vi "TangensFilter3.vi"(4 "error IN":errorcluster, 5 "Max Angle REVERSE Disp":dbl, 6 "Max Angle FORWARD Displ":dbl, 7 "Finded Chains (X,Y,dX,dY)":dbl[][](array[numeric])) -> (0 "error out":errorcluster, 1 "Filtered Chains (X,Y,dX,dY)":dbl[][](array[numeric]), 2 "Saved Chains":i32, 3 "Angles OUT":dbl[][](array[numeric]))   [LabVIEW 2013]
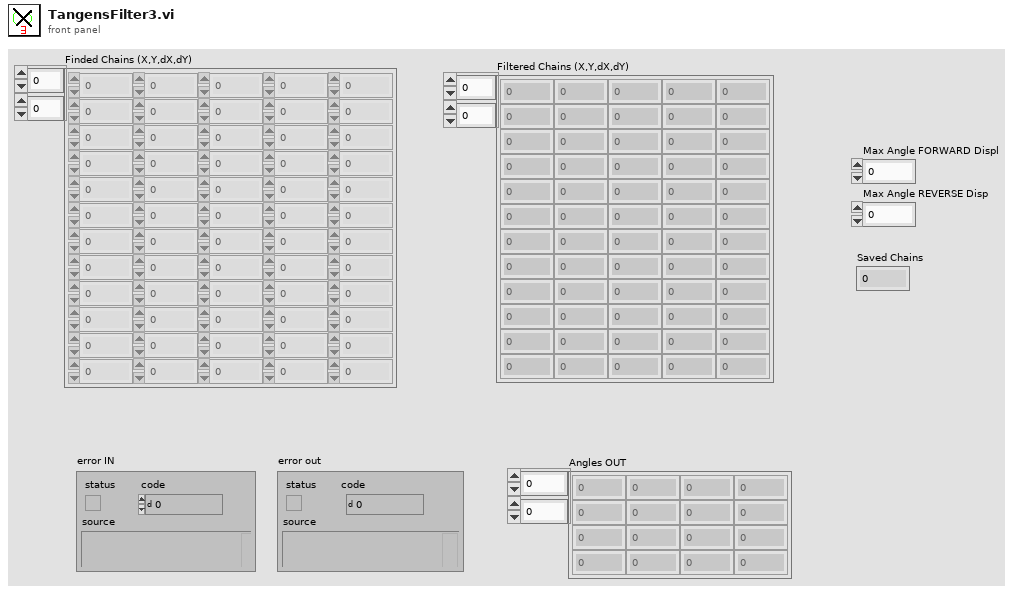
[diagram p1: front panel]
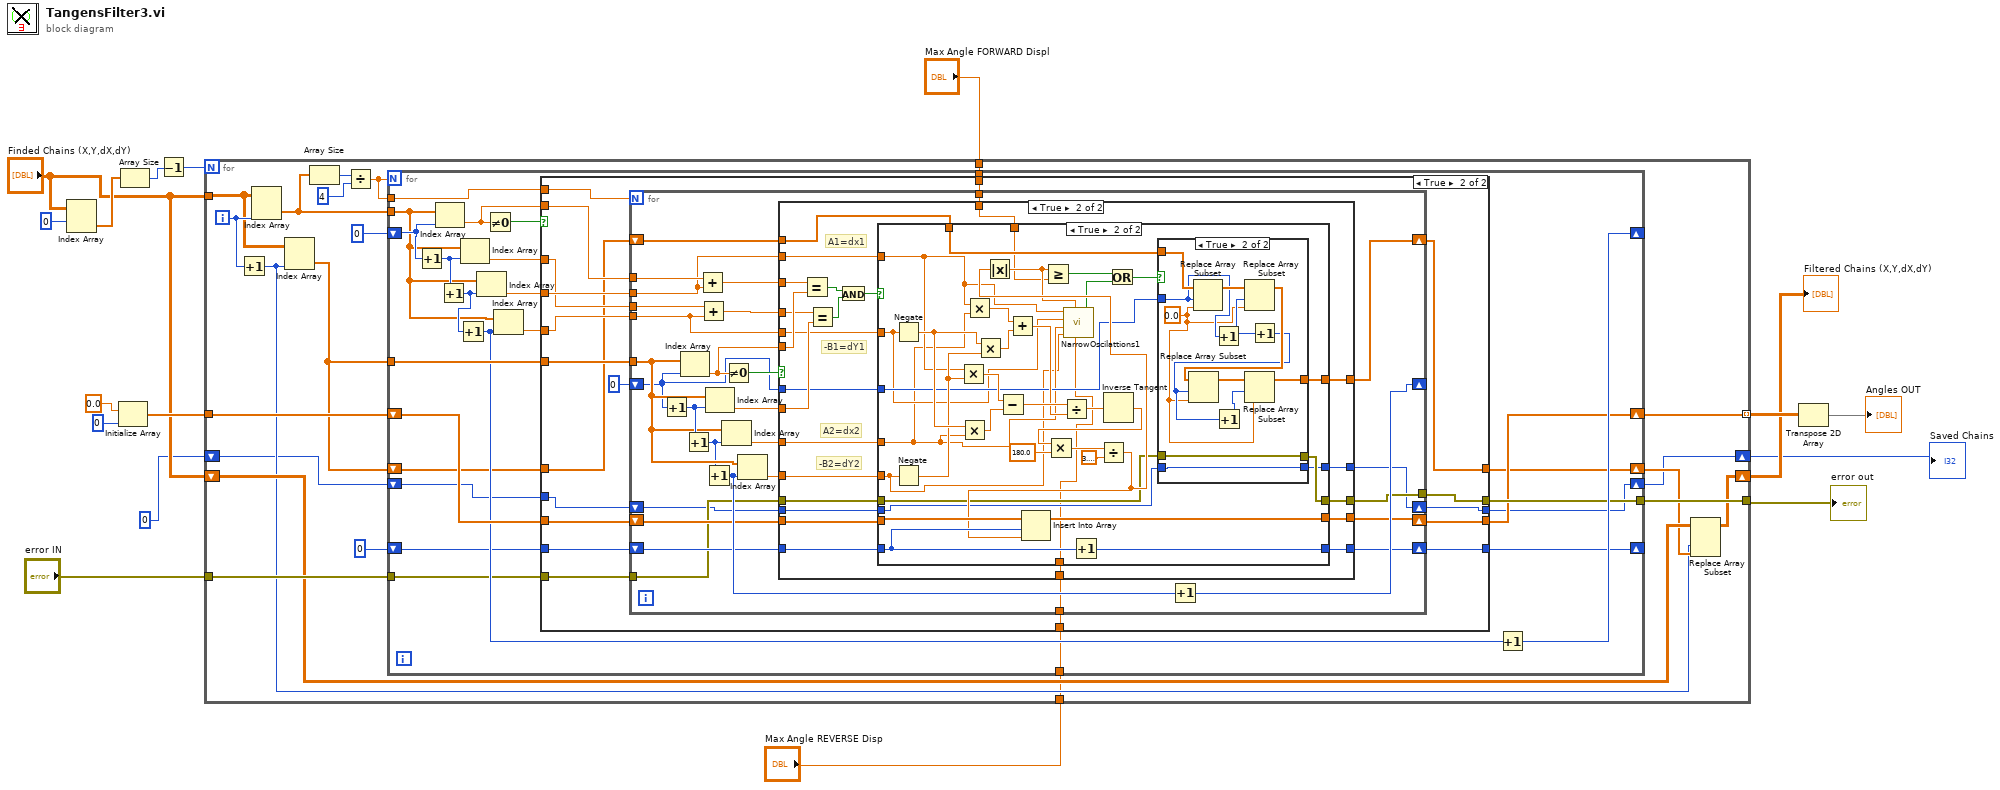
[diagram p0: block diagram]
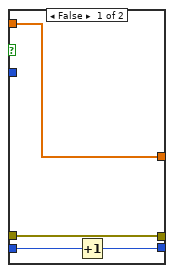
[diagram p5: hidden frame]
diagram:
  n1 = Index Array(array="Finded Chains (X,Y,dX,dY)", index (row)=0 ("disabled index (col)")) -> (element=w16:dbl[])  [unwired: 1 in]
  n2 = Initialize Array(0.0 ("element"), 0 ("dimension size")) -> (w11:dbl[])
  n3 = Array Size(array=w16) -> (size(s)=w15:i32)
  n4 = Decrement(x=w15) -> (x-1=w14:i32)
  n5 = for {
    N: w14 -> [_]
    tunnel: "Finded Chains (X,Y,dX,dY)" -> [w32]
    tunnel: w11 -> [w31]
    tunnel: "error IN" -> [w30]
    tunnel: [w29] -> w9
    tunnel: [w28] -> w8 mode=indexing
    shift-right: [w22] -> w5
    shift-left: "Finded Chains (X,Y,dX,dY)" -> [w25]
    shift-right: [w20] -> w3
    shift-left: 0 -> [w21]
    tunnel: "Max Angle FORWARD Displ" -> [w19]
    tunnel: "Max Angle REVERSE Disp" -> [w18]
    i -> [w33]
    n6 = Increment(x=w33) -> (x+1=w23:i32)
    n7 = Index Array(array=w32, index (col)=w33) -> (element=w36:dbl[])  [unwired: 1 in]
    n8 = Index Array(array=w32, index (col)=w23) -> (element=w26:dbl[])  [unwired: 1 in]
    n9 = Array Size(array=w36) -> (size(s)=w38:i32)
    n10 = Divide(x=w38, y=4) -> (x/y=w34:dbl)
    n11 = for {
      N: w34 -> [_]
      tunnel: w36 -> [w60]
      shift-right: [w51] -> _
      shift-left: 0 -> [w63]
      tunnel: w34 -> [w58]
      shift-right: [w47] -> w28
      shift-left: w31 -> [w53]
      tunnel: w26 -> [w52]
      tunnel: w30 -> [w49]
      tunnel: [w48] -> w29
      shift-right: [w45] -> _
      shift-left: 0 -> [w46]
      shift-right: [w43] -> w24
      shift-left: w26 -> [w44]
      shift-right: [w41] -> w20
      shift-left: w21 -> [w42]
      tunnel: w19 -> [w40]
      tunnel: w18 -> [w39]
      n12 = Increment(x=w63) -> (x+1=w62:i32)
      n13 = Index Array(array=w60, index=w63) -> (element=w57:dbl)
      n14 = Increment(x=w62) -> (x+1=w61:i32)
      n15 = Increment(x=w61) -> (x+1=w50:i32)
      n16 = Index Array(array=w60, index=w62) -> (element=w56:dbl)
      n17 = Index Array(array=w60, index=w61) -> (element=w55:dbl)
      n18 = Not Equal To 0?(x=w57) -> (x != 0?=w59:bool)
      n19 = Index Array(array=w60, index=w50) -> (element=w54:dbl)
      n20 = case shown="True" w59 {
        tunnel: w58 -> [_ w87]
        tunnel: w57 -> [_ w82]
        tunnel: w56 -> [_ w80]
        tunnel: w55 -> [_ w81]
        tunnel: w54 -> [_ w79]
        tunnel: w53 -> [w67 w86]
        tunnel: w52 -> [_ w85]
        tunnel: w49 -> [w68 w83]
        tunnel: w46 -> [w66 w78]
        tunnel: [w68 w77] -> w48
        tunnel: [w67 w76] -> w47
        tunnel: [w66 w75] -> w45
        tunnel: w44 -> [w65 w74]
        tunnel: [w65 w73] -> w43
        tunnel: w42 -> [w64 w72]
        tunnel: [w64 w71] -> w41
        tunnel: w40 -> [_ w70]
        tunnel: w39 -> [_ w69]
        frame False {
        }
        frame True {
          n21 = for {
            N: w87 -> [_]
            tunnel: w85 -> [w115]
            shift-right: [w112] -> _
            shift-left: 0 -> [w93]
            shift-right: [w98] -> w76
            shift-left: w86 -> [w104]
            tunnel: w83 -> [w96]
            tunnel: w82 -> [w110]
            tunnel: w81 -> [w103]
            tunnel: w80 -> [w109]
            tunnel: w79 -> [w102]
            shift-right: [w97] -> w75
            shift-left: w78 -> [w99]
            tunnel: [w95] -> w77
            shift-right: [w92] -> w73
            shift-left: w74 -> [w94]
            shift-right: [w90] -> w71
            shift-left: w72 -> [w91]
            tunnel: w70 -> [w89]
            tunnel: w69 -> [w88]
            n22 = Increment(x=w93) -> (x+1=w116:i32)
            n23 = Index Array(array=w115, index=w93) -> (element=w107:dbl)
            n24 = Increment(x=w116) -> (x+1=w114:i32)
            n25 = Add(x=w110, y=w103) -> (x+y=w108:dbl)
            n26 = Add(x=w109, y=w102) -> (x+y=w106:dbl)
            n27 = Increment(x=w114) -> (x+1=w113:i32)
            n28 = Index Array(array=w115, index=w116) -> (element=w105:dbl)
            n29 = Index Array(array=w115, index=w114) -> (element=w101:dbl)
            n30 = Not Equal To 0?(x=w107) -> (x != 0?=w111:bool)
            n31 = Index Array(array=w115, index=w113) -> (element=w100:dbl)
            n32 = case shown="True" w111 {
              tunnel: w108 -> [_ w145]
              tunnel: w107 -> [_ w144]
              tunnel: w106 -> [_ w143]
              tunnel: w105 -> [_ w142]
              tunnel: w104 -> [w120 w138]
              tunnel: w103 -> [_ w137]
              tunnel: w102 -> [_ w136]
              tunnel: w101 -> [_ w135]
              tunnel: w100 -> [_ w134]
              tunnel: w99 -> [w119 w133]
              tunnel: [w120 w132] -> w98
              tunnel: [w119 w131] -> w97
              tunnel: w96 -> [w121 w130]
              tunnel: [w121 w129] -> w95
              tunnel: w94 -> [w118 w128]
              tunnel: w93 -> [_ w127]
              tunnel: [w118 w126] -> w92
              tunnel: w91 -> [w117 w125]
              tunnel: [w117 w124] -> w90
              tunnel: w89 -> [_ w123]
              tunnel: w88 -> [_ w122]
              frame False {
              }
              frame True {
                # "-B2=dY2"
                # "A2=dx2"
                # "-B1=dY1"
                # "A1=dx1"
                n33 = Equal?(x=w145, y=w144) -> (x = y?=w141:bool)
                n34 = Equal?(x=w143, y=w142) -> (x = y?=w140:bool)
                n35 = And(x=w141, y=w140) -> (x .and. y?=w139:bool)
                n36 = case shown="True" w139 {
                  tunnel: w138 -> [w150 w172]
                  tunnel: w137 -> [_ w159]
                  tunnel: w136 -> [_ w158]
                  tunnel: w135 -> [_ w157]
                  tunnel: w134 -> [_ w156]
                  tunnel: w133 -> [w149 w170]
                  tunnel: [w150 w171] -> w132
                  tunnel: [w149 w169] -> w131
                  tunnel: w130 -> [w148 w164]
                  tunnel: [w148 w163] -> w129
                  tunnel: w128 -> [w147 w167]
                  tunnel: w127 -> [_ w166]
                  tunnel: [w147 w165] -> w126
                  tunnel: w125 -> [w146 w162]
                  tunnel: [w146 w161] -> w124
                  tunnel: w123 -> [_ w152]
                  tunnel: w122 -> [_ w151]
                  frame False {
                  }
                  frame True {
                    n37 = Negate(x=w158) -> (-x=w183:dbl)
                    n38 = Negate(x=w156) -> (-x=w182:dbl)
                    n39 = Multiply(x=w159, y=w182) -> (x*y=w185:dbl)
                    n40 = Multiply(x=w183, y=w157) -> (x*y=w184:dbl)
                    n41 = Multiply(x=w159, y=w157) -> (x*y=w181:dbl)
                    n42 = Multiply(x=w183, y=w182) -> (x*y=w180:dbl)
                    n43 = Subtract(x=w185, y=w184) -> (x-y=w179:dbl)
                    n44 = Add(x=w181, y=w180) -> (x+y=w178:dbl)
                    n45 = Divide(x=w179, y=w178) -> (x/y=w177:dbl)
                    n46 = Increment(x=w170) -> (x+1=w169:i32)
                    n47 = Inverse Tangent(1:w177) -> (0:w176:dbl)
                    n48 = Multiply(x=w176, y=180.0) -> (x*y=w174:dbl)
                    n49 = Divide(x=w174, y=3.141592653589793) -> (x/y=w168:dbl)
                    n50 = Absolute Value(x=w168) -> (abs(x)=w160:dbl)
                    n51 = Insert Into Array(array=w172, index=w170, new element=w168) -> (w171:dbl[])
                    n52 = Greater Or Equal?(x=w160, y=w152) -> (x >= y?=w155:bool)
                    n53 = call "NarrowOscilattions1.vi"("Max Angle"=w151, "Angle"=w160, "dY2"=w156, "dX2"=w157, "dY1"=w158, "dX1"=w159) -> ("Backward Displacement!"=w154:bool)
                    n54 = Or(x=w155, y=w154) -> (x .or. y?=w153:bool)
                    n55 = case shown="True" w153 {
                      tunnel: w167 -> [w189 w201]
                      tunnel: w166 -> [_ w199]
                      tunnel: [w189 w192] -> w165
                      tunnel: [w188 w191] -> w163
                      tunnel: w164 -> [w188 w191]
                      tunnel: [w186 w190] -> w161
                      tunnel: w162 -> [w187 w190]
                      frame False {
                        n56 = Increment(x=w187) -> (x+1=w186:i32)
                      }
                      frame True {
                        w193 = 0.0 ("new element/subarray")
                        n57 = Replace Array Subset(array=w201, new element=w193, index=w199) -> (w200:dbl[])
                        n58 = Increment(x=w199) -> (x+1=w197:i32)
                        n59 = Replace Array Subset(array=w200, new element=w193, index=w197) -> (w198:dbl[])
                        n60 = Increment(x=w197) -> (x+1=w195:i32)
                        n61 = Replace Array Subset(array=w198, new element=w193, index=w195) -> (w196:dbl[])
                        n62 = Increment(x=w195) -> (x+1=w194:i32)
                        n63 = Replace Array Subset(array=w196, new element=w193, index=w194) -> (w192:dbl[])
                      }
                    }
                  }
                }
              }
            }
            n64 = Increment(x=w113) -> (x+1=w112:i32)
          }
        }
      }
      n65 = Increment(x=w50) -> (x+1=w51:i32)
    }
    n66 = Replace Array Subset(array=w25, new element=w24, index (col)=w23) -> (w22:dbl[][])  [unwired: 1 in]
  }
  "error out" <- w9
  "Filtered Chains (X,Y,dX,dY)" <- w5
  "Saved Chains" <- w3
  n67 = Transpose 2D Array(2D array=w8) -> (transposed array=→"Angles OUT":dbl[][])
